vi "Init UI.vi"(8 "error in (no error)":errorcluster, 11 "Deck in":refnum<class "Sample.lvclass">) -> (0 "error out":errorcluster, 3 "Deck out":refnum<class "Sample.lvclass">)   [LabVIEW 2020, in "Sample.lvclass"]
uses:
  Sample.lvclass
  Sample.lvclass/Sample.ctl
  Packed Libraries/Messaging.lvlibp
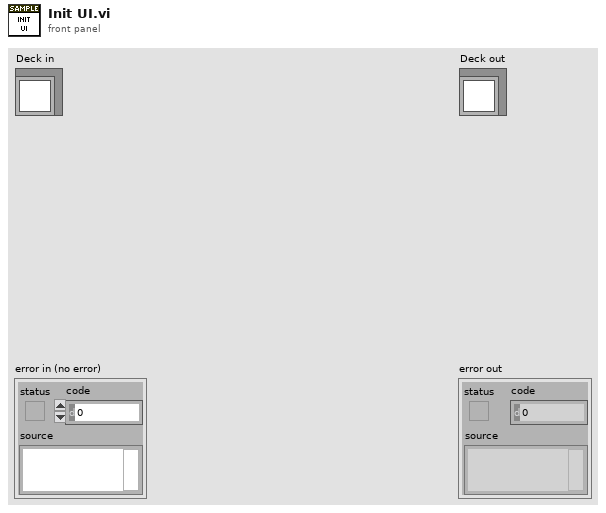
[diagram p1: front panel]
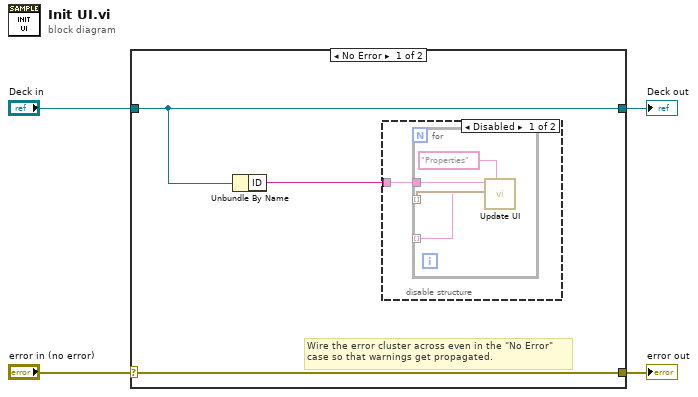
[diagram p0: block diagram]
diagram:
  n1 = case shown="No Error" "error in (no error)" {
    selector: "error in (no error)" -> [w7 w14]
    tunnel: [w7 w14] -> w3
    tunnel: [w6 w13] -> w1
    tunnel: "Deck in" -> [w6 w13]
    frame No Error {
      # "Wire the error cluster across even in the \"No Error\"\ncase so that warnings get propagated."
      n2 = Unbundle By Name(w6) -> ("ID"=w5:string)
      n3 = disable-structure shown="Disabled" {
        disable-tunnel: w5 -> [w8 _]
        frame Disabled {
          n4 = for {
            tunnel: w8 -> [w12]
            tunnel: _ -> [w11] mode=indexing
            tunnel: _ -> [w10] mode=indexing
            n5 = call "Update UI.vi"("Message (Value Change)"="Properties", "Data"=w11, "Target"=w10, "ID"=w12) -> ()  [unwired: 7 in, 1 out]
          }
        }
        frame Enabled {
        }
      }
    }
    frame Error {
    }
  }
  "error out" <- w3
  "Deck out" <- w1
